vi "Set Columns.vi"(3 "error in (no error)":errorcluster, 4 "Columns":refnum<class "Column.lvclass">[](array[class]), 5 "NI Card in":refnum<class "NI Card.lvclass">) -> (0 "error out":errorcluster, 1 "NI Card out":refnum<class "NI Card.lvclass">)   [LabVIEW 2013, in "NI Card.lvclass"]
uses:
  NI Card.lvclass
  ColumnVIs/Column/Column.lvclass
  NI Card.lvclass/NI Card.ctl
  <vilib>/Utility/error.llb/DialogType.ctl
  Device/Device.lvclass
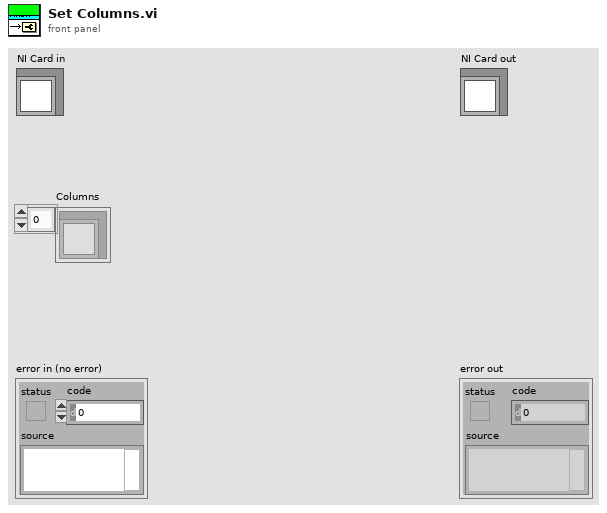
[diagram p1: front panel]
types:
  T1 = cluster{"DAQmx Global Channel":refnum<k21>, "String":string}[]
  T2 = typedef "DialogType.ctl" = u16
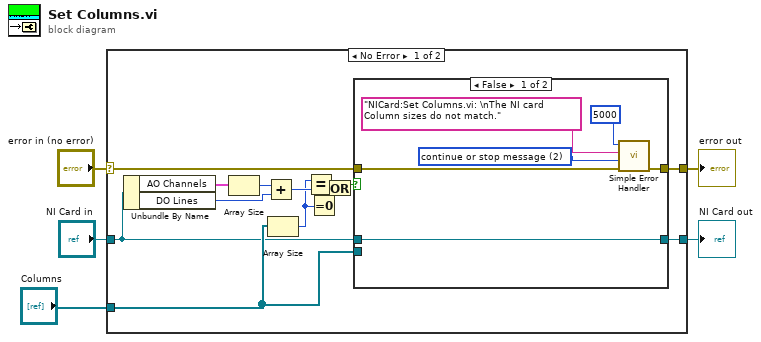
[diagram p0: block diagram]
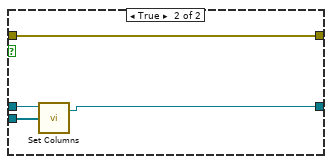
[diagram p2: hidden frame]
diagram:
  n1 = case shown="No Error" "error in (no error)" {
    selector: "error in (no error)" -> [w17 w29]
    tunnel: [w16 w29] -> w4
    tunnel: "NI Card in" -> [w12 w30]
    tunnel: "Columns" -> [w15 _]
    tunnel: [w18 w30] -> w5
    frame No Error {
      n2 = Unbundle By Name(w12) -> ("AO Channels"=w13:T1, "DO Lines"=w9:i32)
      n3 = Array Size(array=w13) -> (size(s)=w11:i32)
      n4 = Add(x=w11, y=w9) -> (x+y=w10:i32)
      n5 = Array Size(array=w15) -> (size(s)=w6:i32)
      n6 = Equal?(x=w6, y=w10) -> (x = y?=w14:bool)
      n7 = Equal To 0?(x=w6) -> (x = 0?=w7:bool)
      n8 = Or(x=w14, y=w7) -> (x .or. y?=w8:bool)
      n9 = case shown="False" w8 {
        tunnel: w12 -> [w24 w26]
        tunnel: w15 -> [_ w27]
        tunnel: [w24 w25] -> w18
        tunnel: w17 -> [w23 w28]
        tunnel: [w22 w28] -> w16
        frame False {
          w20 = T2 2 items=["no dialog", "OK message", "continue or stop message", "OK message + warnings", "continue/stop + warnings"] ("type of dialog (OK msg:1)")
          n10 = call <vilib>:"Simple Error Handler.vi"("error code (no error:0)"=5000, "error source (\" \")"="NICard:Set Columns.vi: \nThe NI card Column sizes do not match." ("message"), "type of dialog (OK msg:1)"=w20, "error in (no error)"=w23) -> ("error out"=w22:errorcluster)  [unwired: 1 in, 4 out]
        }
        frame True {
          n11 = call-parent "Set Columns.vi"("Columns"=w27, "Device in"=w26) -> ("Device out"=w25:refnum<class "NI Card.lvclass">)  [unwired: 2 in, 1 out]
        }
      }
    }
    frame Error {
    }
  }
  "error out" <- w4
  "NI Card out" <- w5
